vi "test Deploy Scripted System Definition.vi"(8 "error in (no error)":errorcluster, 11 "TestCase in":refnum<class "NI-SWITCH Scripting System Tests.lvclass">=refnum) -> (0 "error out":errorcluster, 3 "TestCase out":refnum<class "NI-SWITCH Scripting System Tests.lvclass">)   [LabVIEW 2017, in "NI-SWITCH Scripting System Tests.lvclass"]
uses:
  NI-SWITCH Scripting System Tests.lvclass
  <vilib>/addons/_JKI Toolkits/VI Tester/TestCase.llb/TestCase.lvclass
  niveristand-custom-device-testing-tools/VeriStandTestCase/VeriStandTestCase.lvclass
  Shared/VeriStand SLSC Scripting/VeriStand SLSC Scripting.lvlib
  NI-SWITCH Scripting.lvlib
  Custom Device/Find SLSC Switch Custom Device by Slot Number.vi
  NationalInstruments.VeriStand.SystemDefinitionAPI
  C:/Dev/GitHub/niveristand-custom-device-testing-tools/VeriStandTestCase/VeriStandTestCase.lvclass
  C:/Program Files (x86)/National Instruments/LabVIEW 2017/vi.lib/addons/_JKI Toolkits/VI Tester/TestCase.llb/TestCase.lvclass
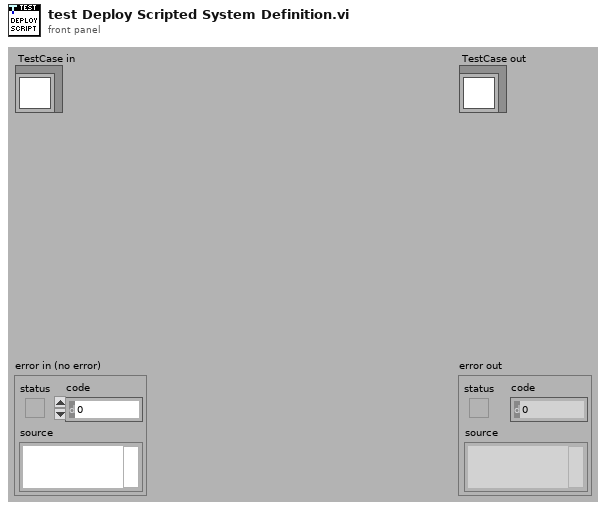
[diagram p1: front panel]
types:
  T1 = typedef "Custom Device API.lvlib/Custom Device Item Ref.ctl" = u64
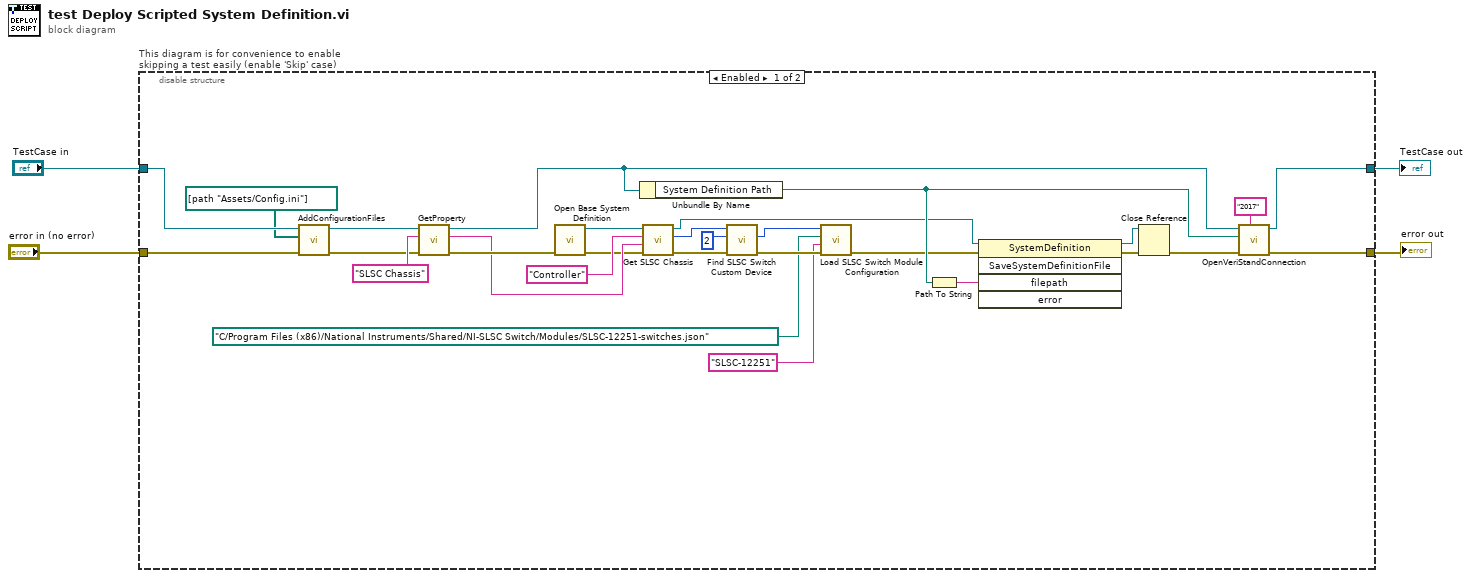
[diagram p0: block diagram]
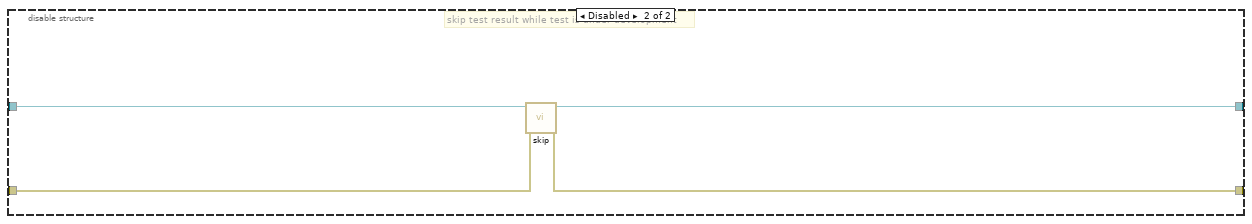
[diagram p2: hidden frame]
diagram:
  n1 = disable-structure "This diagram is for convenience to enable skipping a test easily (enable 'Skip' case)" shown="Enabled" {
    disable-tunnel: "TestCase in" -> [w21 w37]
    disable-tunnel: [w33 w35] -> w1
    disable-tunnel: [w32 w36] -> w3
    disable-tunnel: "error in (no error)" -> [w24 w34]
    frame Enabled {
      n2 = call "AddConfigurationFiles.vi"("error in (no error)"=w24, "configuration files"=path[] [path "Assets/Config.ini"], "VeriStandTestCase in"=w21) -> ("error out"=w23:errorcluster, "VeriStandTestCase out"=w22:refnum<class "NI-SWITCH Scripting System Tests.lvclass">)  [unwired: 7 in]
      n3 = call "GetProperty.vi"("error in (no error)"=w23, "key"="SLSC Chassis", "VeriStandTestCase in"=w22) -> ("error out"=w19:errorcluster, "value"=w6:string, "VeriStandTestCase out"=w18:refnum<class "NI-SWITCH Scripting System Tests.lvclass">)  [unwired: 6 in]
      n4 = call "Open Base System Definition.vi"("error in (no error)"=w19) -> ("error out"=w5:errorcluster, "SystemDefinition"=w9:refnum<k24>)  [unwired: 9 in]
      n5 = Unbundle By Name(w18) -> ("System Definition Path"=w28:path)
      n6 = call "Get SLSC Chassis.vi"("error in (no error)"=w5, "SLSC Chassis Name or IP"=w6, "Target Name"="Controller" ("Target"), "SysDef in"=w9) -> ("error out"=w15:errorcluster, "SLSC Chassis"=w16:u64, "SysDef out"=w8:refnum<k24>)  [unwired: 4 in, 1 out]
      n7 = call-poly "Find SLSC Switch Custom Device.vi"("error in"=w15, "slot number"=2, "slsc chassis in"=w16) -> ("error out"=w17:errorcluster, "slsc switch custom device"=w11:T1)  [unwired: 6 in, 1 out]
      n8 = call "Load SLSC Switch Module Configuration.vi"("error in"=w17, "product name"="SLSC-12251" ("Model"), "switches json file"=path "C:/Program Files (x86)/National Instruments/Shared/NI-SLSC Switch/Modules/SLSC-12251-switches.json" ("switches JSON file"), "slsc switch custom device in"=w11) -> ("error out"=w7:errorcluster)  [unwired: 6 in, 1 out]
      n9 = Path To String(path=w28) -> (string=w29:string)
      n10 = invoke class="SystemDefinition" method="SaveSystemDefinitionFile"(reference=w8, error in=w7, "filepath"=w29) -> (reference out=w30:refnum<k24>, error out=w31:errorcluster)  [unwired: 2 in, 3 out]
      n11 = Close Reference(reference=w30, error in (no error)=w31) -> (error out=w26:errorcluster)
      n12 = call-dynamic "OpenVeriStandConnection.vi"("Minimum VeriStand Version (2016)"="2017" ("Minimum VeriStand Version (2015)"), "error in (no error)"=w26, "System Definition File"=w28, "VeriStand Test Case in"=w18) -> ("error out"=w32:errorcluster, "VeriStand Test Case out"=w33:refnum<class "NI-SWITCH Scripting System Tests.lvclass">)  [unwired: 5 in, 1 out]
    }
    frame Disabled {
      # "skip test result while test is under development"
      n13 = call <vilib>:"skip.vi"("error in (no error)"=w34, "TestCase in"=w37) -> ("error out"=w36:errorcluster, "TestCase out"=w35:refnum<class "NI-SWITCH Scripting System Tests.lvclass">)  [unwired: 8 in]
    }
  }
  "error out" <- w3
  "TestCase out" <- w1
